vi "saveDataNodeBegin.vi"(8 "error in (no error)":errorcluster, 9 "indent":i32, 10 "XML Refnum in":refnum<file>, 11 "Packet in":refnum<class "Packet.lvclass">) -> (0 "error out":errorcluster, 2 "XML Refnum out":refnum<file>, 3 "Packet out":refnum<class "Packet.lvclass">)   [LabVIEW 2013, in "Packet.lvclass"]
doc: "Begins the process of saving a xceData Node to an XML formatted file."
uses:
  Packet.lvclass
  xCE/xceNode/xceNode.lvclass
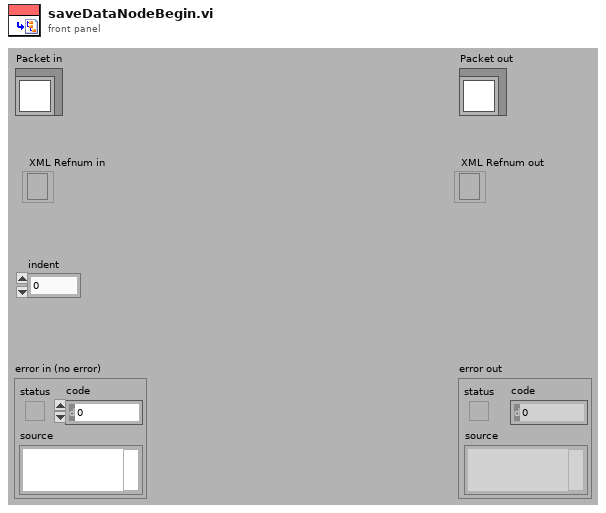
[diagram p1: front panel]
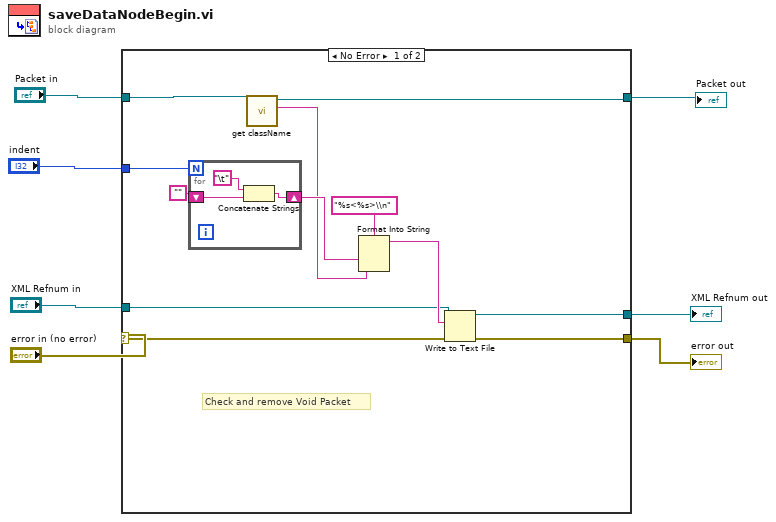
[diagram p0: block diagram]
diagram:
  n1 = case shown="No Error" "error in (no error)" {
    selector: "error in (no error)" -> [w9 w24]
    tunnel: "Packet in" -> [w10 w25]
    tunnel: "indent" -> [w8 _]
    tunnel: [w15 w25] -> w1
    tunnel: [w14 w23] -> w3
    tunnel: [w13 w24] -> w2
    tunnel: "XML Refnum in" -> [w11 w23]
    frame No Error {
      # "Check and remove Void Packet"
      n2 = for {
        N: w8 -> [_]
        shift-right: [w22] -> w18
        shift-left: "" -> [w21]
        n3 = Concatenate Strings("\t", w21) -> (w22:string)
      }
      n4 = call "get className.vi"("xceNode in"=w10) -> ("Class name"=w16:string, "xceNode out"=w15:refnum<class "Packet.lvclass">)  [unwired: 8 in, 1 out]
      n5 = Format Into String(format string="%s<%s>\\n", w18, w16) -> (resulting string=w12:string)  [unwired: 2 in, 1 out]
      n6 = Write to Text File(file (use dialog)=w11, text=w12, error in=w9) -> (refnum out=w14:refnum<file>, error out=w13:errorcluster)  [unwired: 1 in, 1 out]
    }
    frame Error {
    }
  }
  "error out" <- w2
  "Packet out" <- w1
  "XML Refnum out" <- w3
